vi "Write DatabaseRef.vi"(8 "error in (no error)":errorcluster, 10 "Database.lvlib:Database":refnum<class "Database.lvclass">, 11 "Plugin in":refnum<class "Plugin.lvclass">) -> (0 "error out":errorcluster, 3 "Plugin out":refnum<class "Plugin.lvclass">)   [LabVIEW 2015, in "ActorManagement.lvlib" / "Plugin.lvclass"]
uses:
  Plugin.lvclass
  DatabaseManagement/Database.lvclass
  Plugin.lvclass/Plugin.ctl
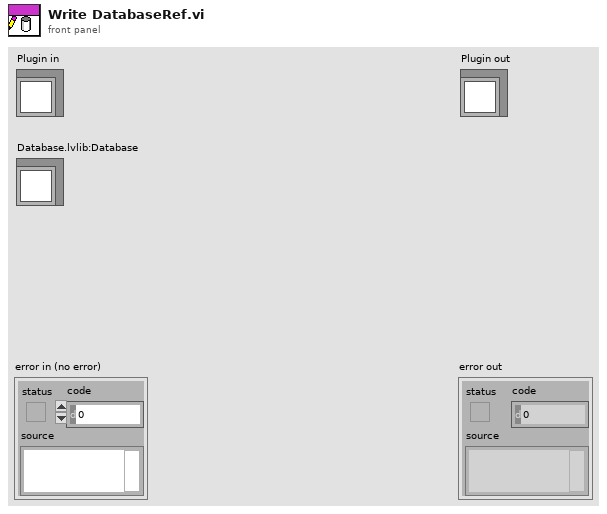
[diagram p1: front panel]
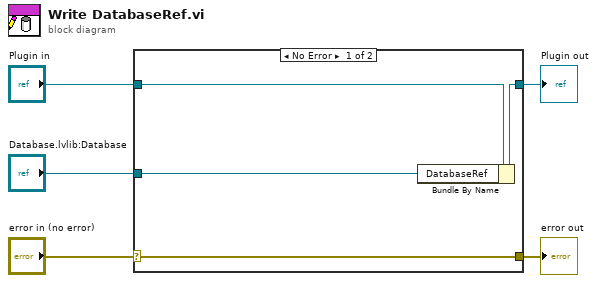
[diagram p0: block diagram]
diagram:
  n1 = case shown="No Error" "error in (no error)" {
    selector: "error in (no error)" -> [w9 w10]
    tunnel: [w9 w10] -> w4
    tunnel: [w7 w11] -> w2
    tunnel: "Plugin in" -> [w8 w11]
    tunnel: "Database.lvlib:Database" -> [w6 _]
    frame No Error {
      n2 = Bundle By Name(cluster=w8, "DatabaseRef"=w6) -> (w7:refnum<class "Plugin.lvclass">)
    }
    frame Error {
    }
  }
  "error out" <- w4
  "Plugin out" <- w2
